vi "FP_Get Pane.vi"(8 "Error":errorcluster, 9 "Pane Index":i32, 11 "VI":refnum<vi>) -> (0 "Error Out":errorcluster, 2 "Pane Refnum Out":refnum<vi>, 3 "VI Out":refnum<vi>)   [LabVIEW 2016]
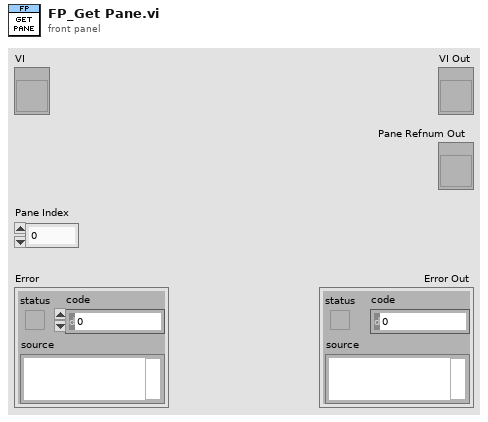
[diagram p1: front panel]
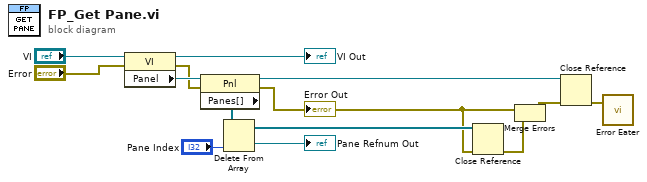
[diagram p0: block diagram]
diagram:
  n1 = property class="VI"(reference="VI", error in="Error") -> (reference out=→"VI Out":refnum<vi>, error out=w6:errorcluster, "Panel"=w8:refnum<vi>)
  n2 = property class="Pnl"(reference=w8, error in=w6) -> (reference out=w9:refnum<vi>, error out=w1:errorcluster, "Panes[]"=w7:refnum<vi>[])
  "Error Out" <- w1
  n3 = Delete From Array(array=w7, index="Pane Index") -> (deleted portion=→"Pane Refnum Out":refnum<vi>, array with subset deleted=w5:refnum<vi>[])  [unwired: 1 in]
  n4 = Close Reference(reference=w5, error in (no error)=w1) -> (error out=w3:errorcluster)
  n5 = Merge Errors(w1, w3) -> (w2:errorcluster)
  n6 = Close Reference(reference=w9, error in (no error)=w2) -> (error out=w4:errorcluster)
  n7 = call "Error Eater.vi"("error in (no error)"=w4) -> ()  [unwired: 2 in]
